vi "Application Memory Monitor.vi"() -> ()   [LabVIEW 2016]
uses:
  <vilib>/Utility/error.llb/DialogType.ctl
  SLL Queued State Machine/Queue Driver/Create Queue.vi
  SLL Queued State Machine/Queue Driver/Enqueue an Item to Queue.vi
  SLL Queued State Machine/Queue Driver/Dequeue Queue.vi
  SLL Queued State Machine/Queue Driver/Enqueue N Items.vi
  SLL Queued State Machine/Queue Driver/Flush Queue.vi
  SLL Queued State Machine/Queue Driver/Release Queue.vi
  SLL Queued State Machine/SLL QSM.lvlib
panel:
  in  "Start":bool
  in  "Sampling Rate (s)":dbl=1.0
  in  "Application Image Name":string="LabVIEW"
  out "Waveform Chart":T1(graph)
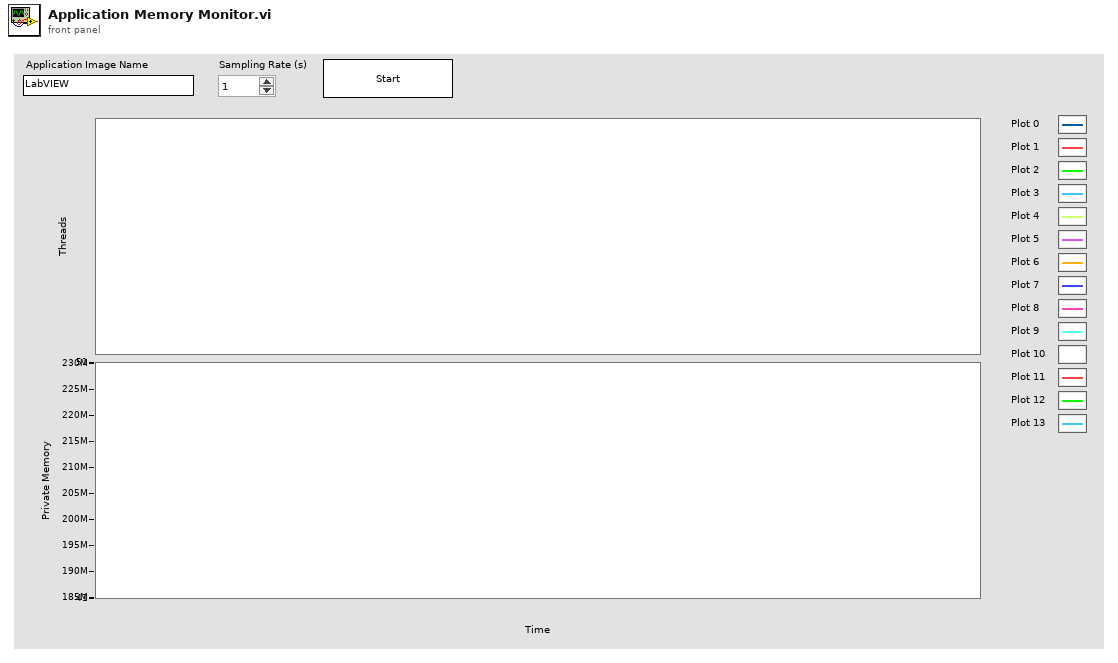
[diagram p1: front panel]
types:
  T1 = cluster{"Thread Count":i32, "PrivateMemorySize64":i64}
  T2 = cluster{"Flags":cluster{"Source Code?":bool, "Running?":bool}, "Application Name":string, "Ref":cluster{"ProcessMain":refnum<k24>, "UserProcess":refnum<k24>, "Threads":refnum<k24>}, "Sampling Rate (ms)":i32}
  T3 = cluster{"Thread Count":i32, "PrivateMemorySize64":i64}[]
  T4 = typedef "DialogType.ctl" = u16
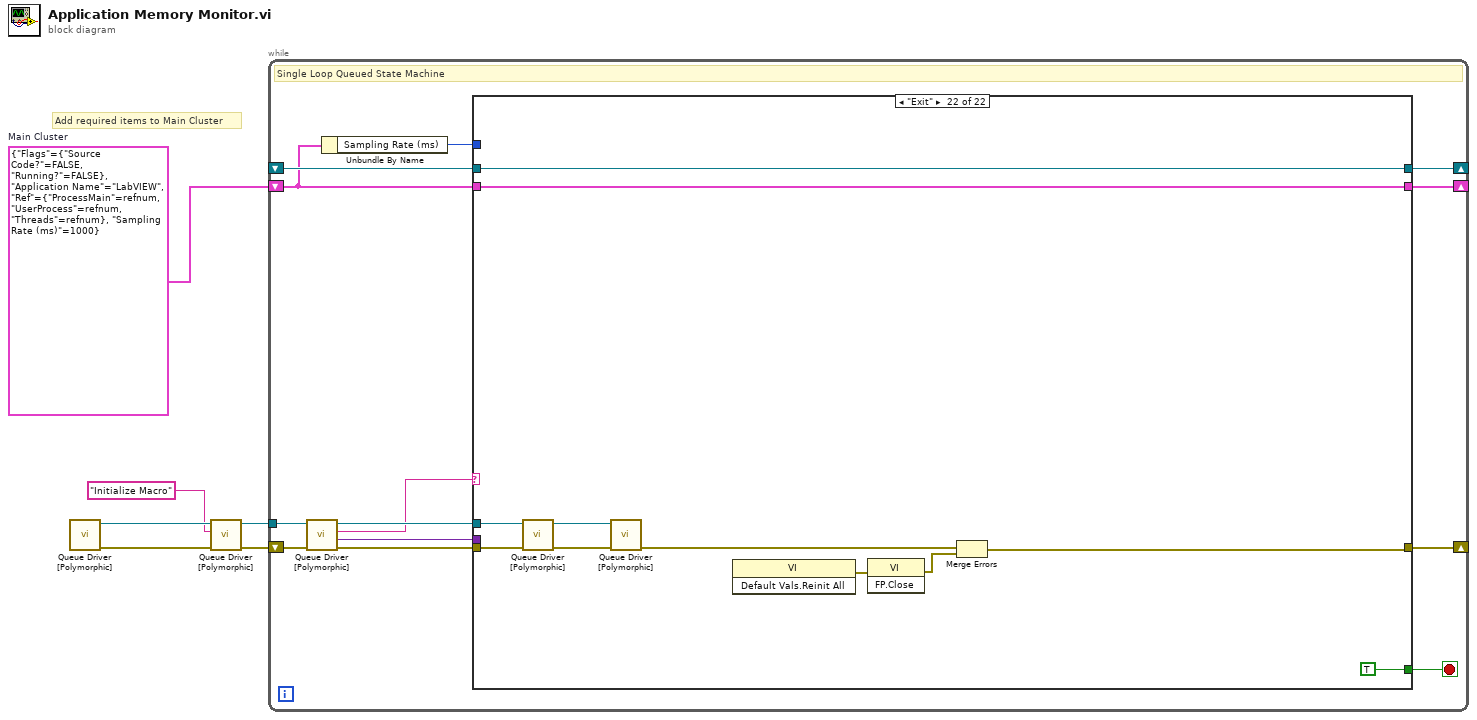
[diagram p0: block diagram]
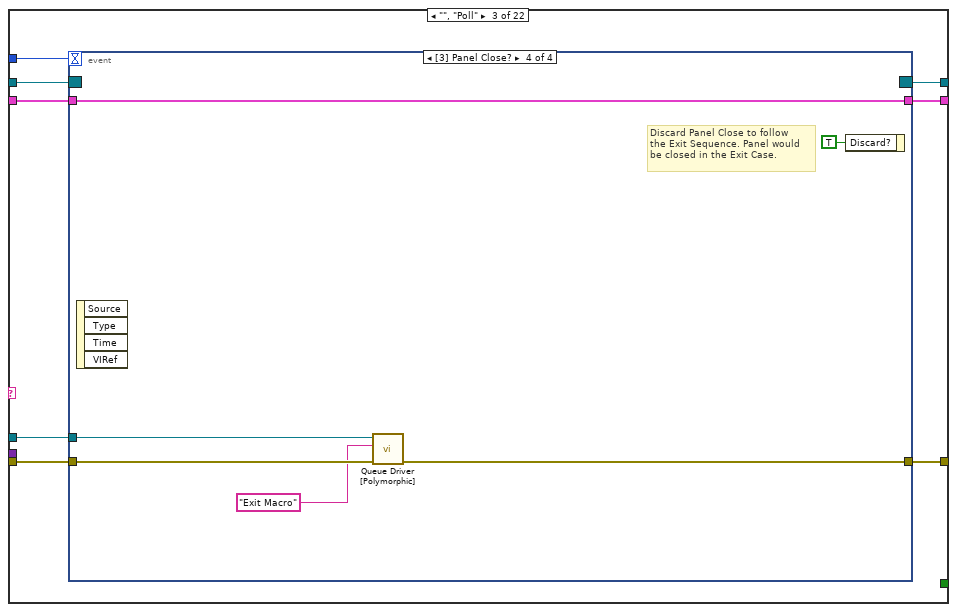
[diagram p4: hidden frame]
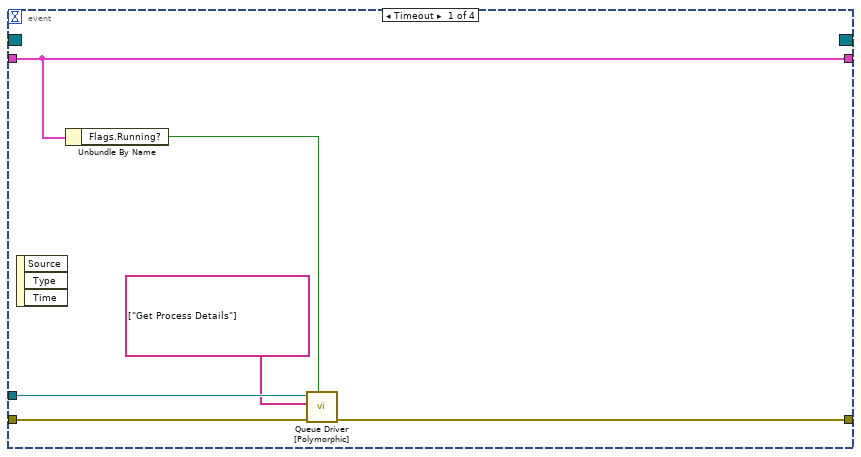
[diagram p5: hidden frame]
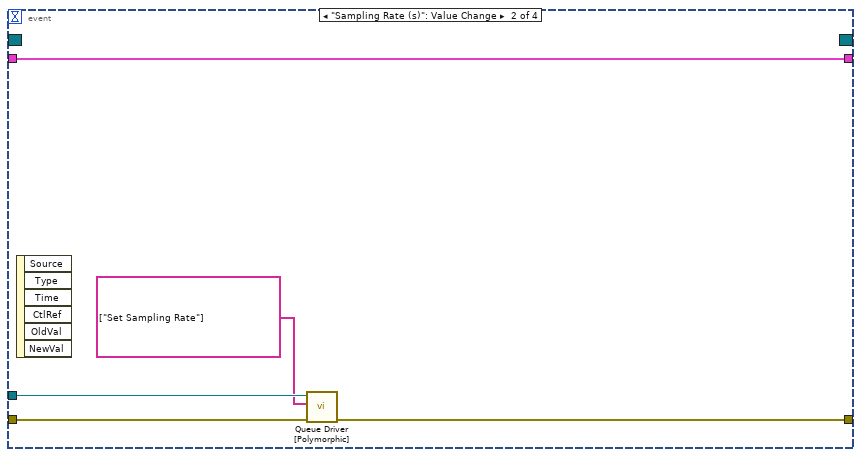
[diagram p6: hidden frame]
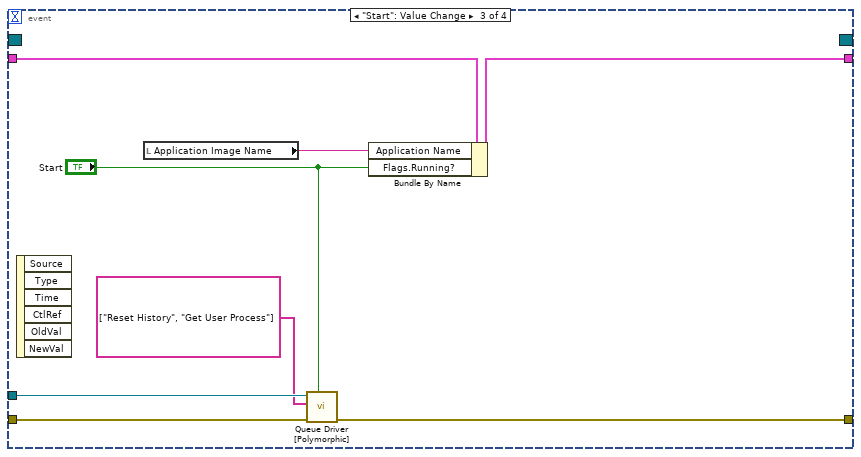
[diagram p7: hidden frame]
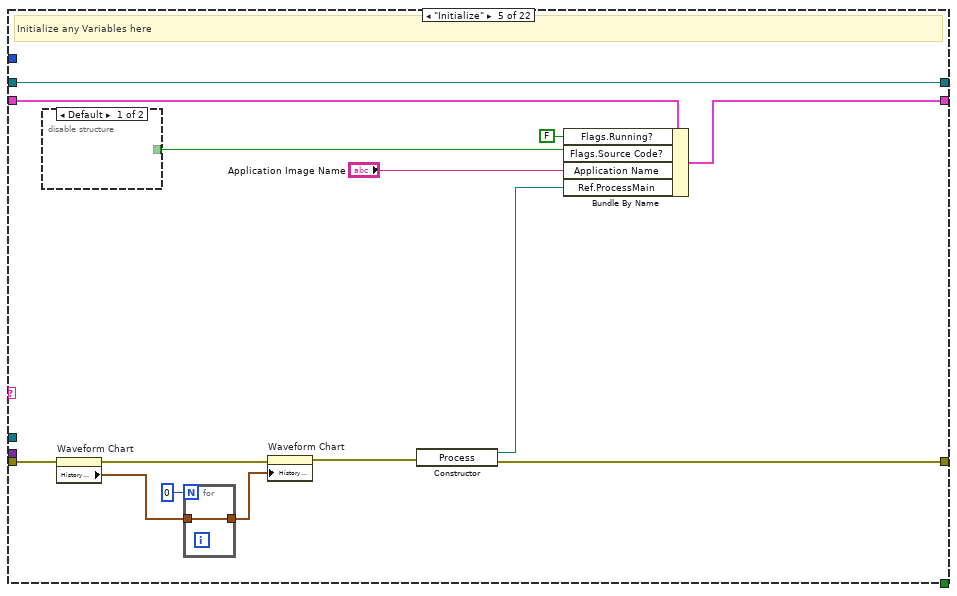
[diagram p9: hidden frame]
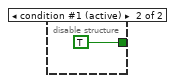
[diagram p10: hidden frame]
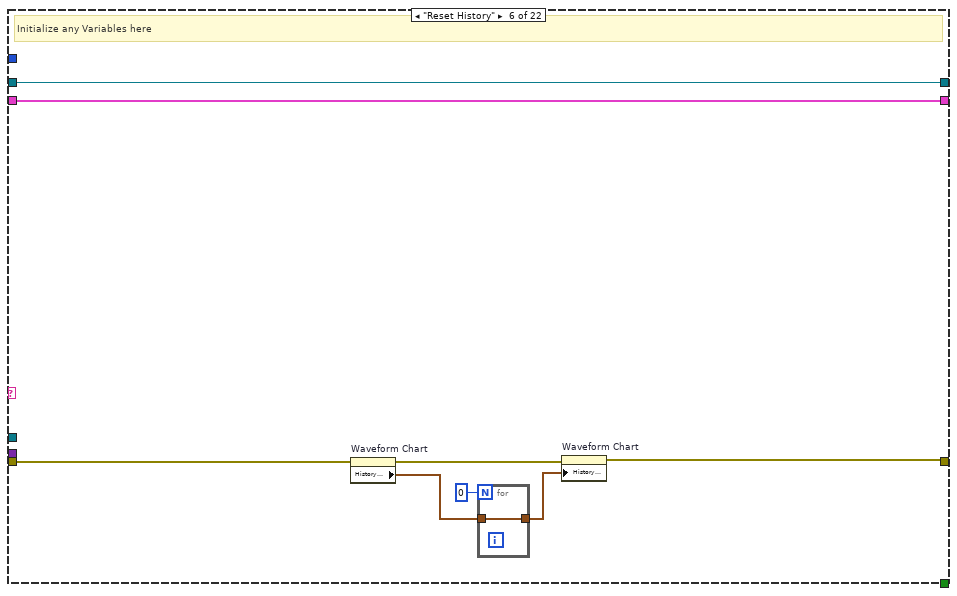
[diagram p11: hidden frame]
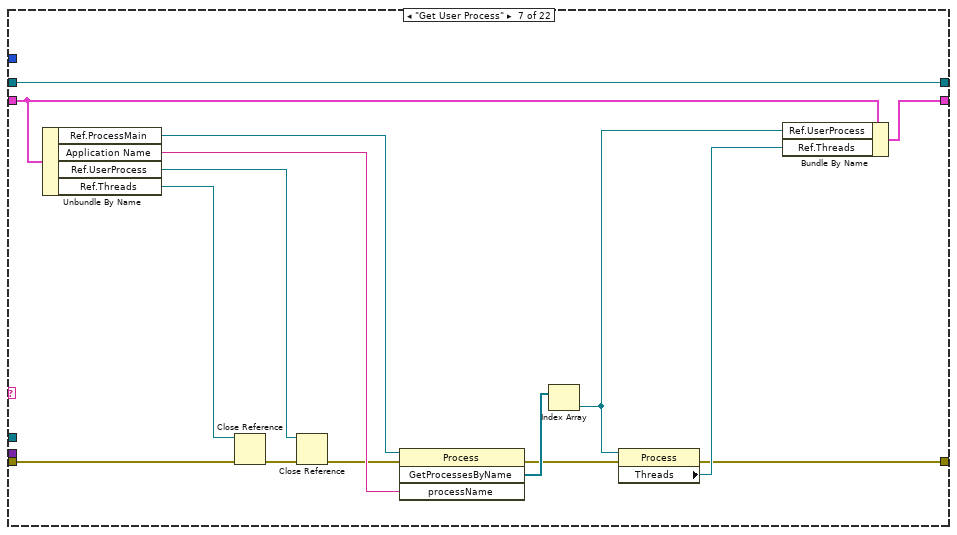
[diagram p12: hidden frame]
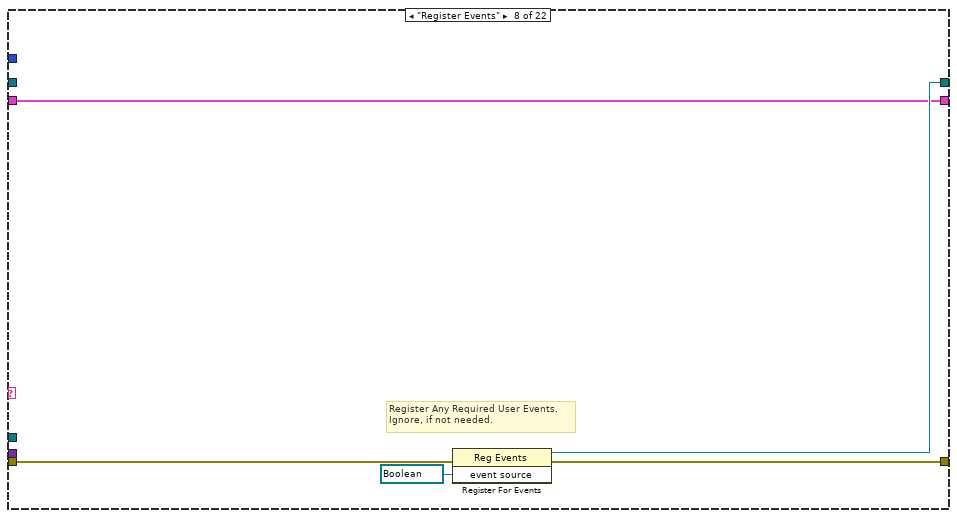
[diagram p13: hidden frame]
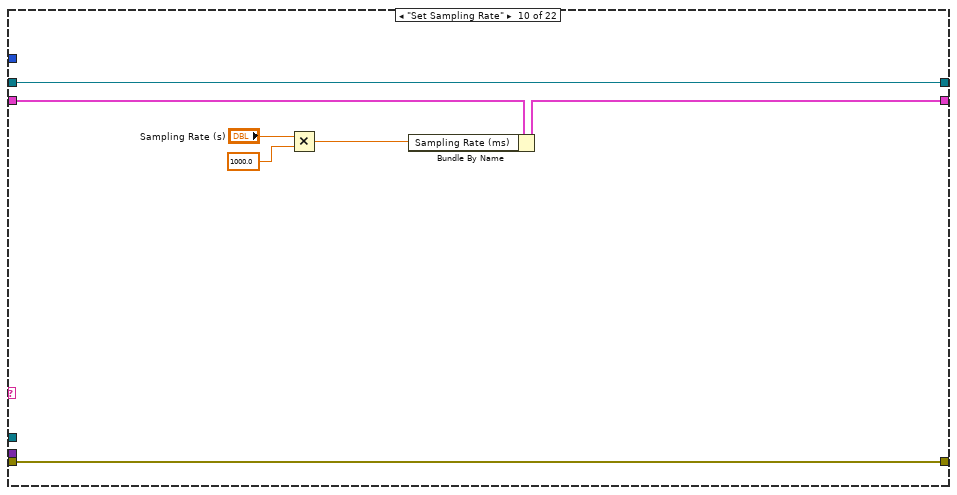
[diagram p15: hidden frame]
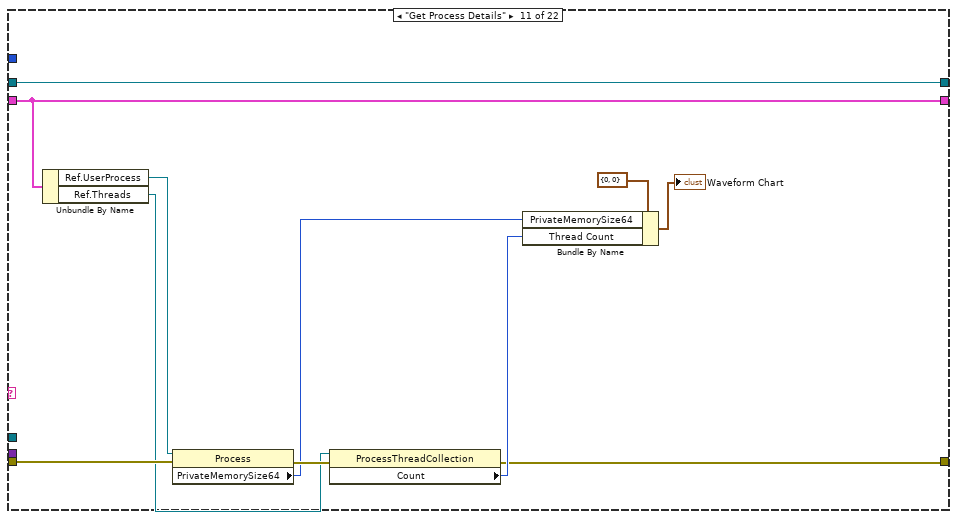
[diagram p16: hidden frame]
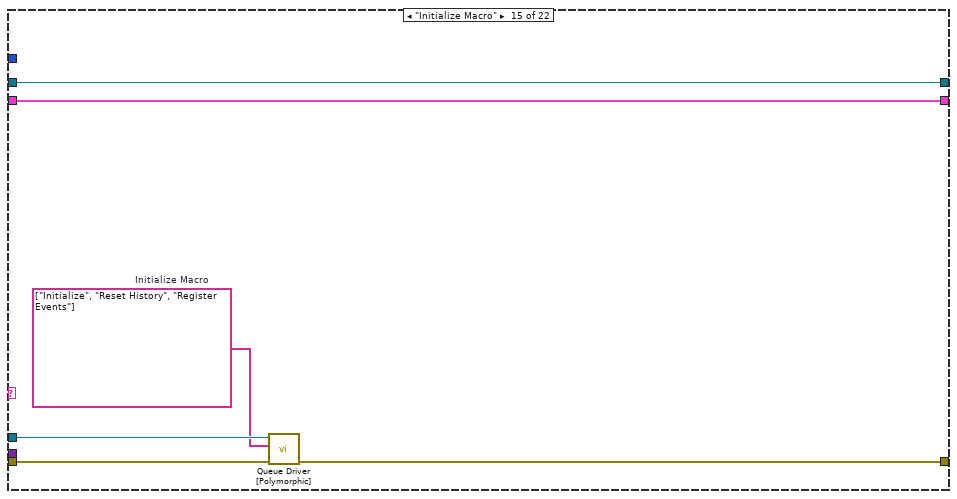
[diagram p20: hidden frame]
diagram:
  w6 = T2 {"Flags"={"Source Code?"=FALSE, "Running?"=FALSE}, "Application Name"="LabVIEW", "Ref"={"ProcessMain"=refnum, "UserProcess"=refnum, "Threads"=refnum}, "Sampling Rate (ms)"=1000}  # Main Cluster
  # "Add required items to Main Cluster"
  n1 = call-poly "Queue Driver [Polymorphic].vi"() -> ("Error Out"=w4:errorcluster, "Queue Ref"=w3:refnum<queue>)  [unwired: 10 in]
  n2 = call-poly "Queue Driver [Polymorphic].vi"("Error In"=w4, "Item to Add"="Initialize Macro", "Queue Ref In"=w3) -> ("Error Out"=w5:errorcluster, "Queue Ref Out"=w1:refnum<queue>)  [unwired: 7 in]
  n3 = while "SLL Queued State Machine" {
    shift-right: [w17] -> _
    shift-left: w5 -> [w19]
    shift-right: [w14] -> _
    shift-left: _ -> [w13]
    shift-right: [w12] -> _
    shift-left: w6 -> [w10]
    tunnel: w1 -> [w8]
    stop <- w16 stop-if-true
    # "Single Loop Queued State Machine"
    n4 = call-poly "Queue Driver [Polymorphic].vi"("Error In"=w19, "Queue Ref In"=w8) -> ("Error Out"=w18:errorcluster, "Data"=w7:variant, "Dequeue"=w11:string, "Queue Ref Out"=w15:refnum<queue>)  [unwired: 6 in]
    n5 = Unbundle By Name(w10) -> ("Sampling Rate (ms)"=w9:i32)
    n6 = case "QSM Case Structure" shown="\"Exit\"" w11 {
      selector: w11 -> [_ _ _ _ _ _ _ _ _ _ _ _ _ _ _ _ _ w152 _ _ _ _]
      tunnel: w18 -> [w22 w25 w32 w61 w68 w83 w98 w106 w109 w116 w125 w130 w133 w136 w140 w146 w151 w155 w167 w170 w174 w188]
      tunnel: [w22 w25 w33 w61 w70 w81 w92 w105 w109 w116 w117 w130 w133 w136 w139 w145 w151 w158 w165 w170 w173 w184] -> w17
      tunnel: [_ _ _ _ _ _ _ _ _ _ _ _ _ _ _ _ _ _ _ _ _ TRUE] -> w16
      tunnel: [w21 w24 w31 w60 w75 w85 w101 w104 w108 w115 w127 w129 w132 w135 w142 w148 w150 w161 w164 w169 w179 w187] -> w14
      tunnel: w13 -> [w21 w24 w30 w60 w75 w85 w101 _ w108 w115 w127 w129 w132 w135 w142 w148 w150 w161 w164 w169 w179 w187]
      tunnel: [w20 w23 w28 w59 w72 w84 w95 w103 w107 w111 w126 w128 w131 w134 w141 w147 w149 w160 w163 w168 w178 w186] -> w12
      tunnel: w10 -> [w20 w23 w29 w59 w73 w84 w96 w103 w107 w114 w126 w128 w131 w134 w141 w147 w149 w160 w163 w168 w178 w186]
      tunnel: w9 -> [_ _ w27 _ _ _ _ _ _ _ _ _ _ _ _ _ _ _ _ _ _ _]
      tunnel: w15 -> [_ _ w26 _ _ _ _ _ _ _ _ _ _ _ w138 w144 _ _ _ _ _ w183]
      tunnel: w7 -> [_ _ _ _ _ _ _ _ _ _ _ _ _ _ _ _ _ _ _ _ _ _]
      frame "/--------------- Read Me -----------------/" {
        # "General Purpose Queue Based State Machine for Any Use Case (main application, module, pop up message etc)\n\nAdvantages:\n1. No Need to Pass Queue References between Queue Driver VIs.\n2. This template can be safely used in multiple parallel running modules without any issues.\n3. This template can also be safely used even in cases where the VI is configured to be a Clone, where multiple \ninstances of the VI could be executing concurrently.\n\nHow to Use:\n1. Add necessary items to the Main Cluster.\n2. Use the Polymorphic Queue Driver for doing any queue operations. There is no need to pass the queue driver\nreference, as the Queue Driver automatically infers the reference based on the VI instance from which it is called.\n3. Add any required user events in the \"Register Events\" case. Ignore if not needed.\n4. Use \"Sequences\" section for defining any list of state calls, which could be used in multiple places. \nExample: Initialize Sequence, might be needed if we need to any reinitialization."
      }
      frame "/------------------ Poll -------------------/" {
      }
      frame "", "Poll" {
        n7 = event shown="[3] Panel Close?" {
          selector: w30 -> [_ _ _ _]
          dyn-events: [_ _ _ _] -> w31
          timeout: w27 -> [_ _ _ _]
          tunnel: [w38 w42 w50 w57] -> w33
          tunnel: w32 -> [w39 w43 w51 w58]
          tunnel: w29 -> [w35 w44 w52 w56]
          tunnel: [w35 w44 w47 w56] -> w28
          tunnel: w26 -> [w37 w41 w49 w53]
          event Timeout {
            n8 = event-data() -> ()  [unwired: 1 in, 3 out]
            n9 = Unbundle By Name(w35) -> ("Flags.Running?"=w34:bool)
            n10 = call-poly "Queue Driver [Polymorphic].vi"("Add to Queue? (T)"=w34, "Error In"=w39, "Enqueue N"=string[] ["Get Process Details"], "Queue Ref In"=w37) -> ("Error Out"=w38:errorcluster)  [unwired: 6 in, 1 out]
          }
          event "Sampling Rate (s)": Value Change {
            n11 = event-data() -> ()  [unwired: 1 in, 6 out]
            n12 = call-poly "Queue Driver [Polymorphic].vi"("Error In"=w43, "Enqueue N"=string[] ["Set Sampling Rate"], "Queue Ref In"=w41) -> ("Error Out"=w42:errorcluster)  [unwired: 7 in, 1 out]
          }
          event "Start": Value Change {
            n13 = event-data() -> ()  [unwired: 1 in, 6 out]
            n14 = local read "Application Image Name"() -> (w45:string)
            n15 = call-poly "Queue Driver [Polymorphic].vi"("Add to Queue? (T)"="Start", "Error In"=w51, "Enqueue N"=string[] ["Reset History", "Get User Process"], "Queue Ref In"=w49) -> ("Error Out"=w50:errorcluster)  [unwired: 6 in, 1 out]
            n16 = Bundle By Name(cluster=w52, "Application Name"=w45, "Flags.Running?"="Start") -> (w47:T2)
          }
          event Panel Close? {
            # "Discard Panel Close to follow\nthe Exit Sequence. Panel would\nbe closed in the Exit Case."
            n17 = event-data() -> ()  [unwired: 1 in, 4 out]
            n18 = call-poly "Queue Driver [Polymorphic].vi"("Error In"=w58, "Item to Add"="Exit Macro" ("Enqueue"), "Queue Ref In"=w53) -> ("Error Out"=w57:errorcluster)  [unwired: 7 in, 1 out]
            n19 = event-data("Discard?"=TRUE) -> ()  [unwired: 1 in, 1 out]
          }
        }
      }
      frame "/--------------- Initialize -----------------/" {
      }
      frame "Initialize" {
        # "Initialize any Variables here"
        n20 = disable-structure shown="Default" {
          disable-tunnel: [_ TRUE] -> w74
          frame condition #0 {
          }
          frame condition #1 (active) {
          }
        }
        n21 = property on="Waveform Chart" class="WFChart (strict)"(error in=w68) -> (error out=w67:errorcluster, "History Data"=w64:T3)  [unwired: 1 in, 1 out]
        n22 = for {
          N: 0 -> [_]
          tunnel: w64 -> [w76]
          tunnel: [w76] -> w63
        }
        n23 = property on="Waveform Chart" class="WFChart (strict)"(error in=w67, "History Data"=w63) -> (error out=w66:errorcluster)  [unwired: 1 in, 1 out]
        n24 = constructor class="Process"(error in=w66) -> (reference out=w69:refnum<k24>, error out=w70:errorcluster)  [unwired: 2 in, 1 out]
        n25 = Bundle By Name(cluster=w73, "Flags.Running?"=FALSE, "Flags.Source Code?"=w74, "Application Name"="Application Image Name", "Ref.ProcessMain"=w69) -> (w72:T2)
      }
      frame "Reset History" {
        # "Initialize any Variables here"
        n26 = property on="Waveform Chart" class="WFChart (strict)"(error in=w83) -> (error out=w82:errorcluster, "History Data"=w79:T3)  [unwired: 1 in, 1 out]
        n27 = for {
          N: 0 -> [_]
          tunnel: w79 -> [w86]
          tunnel: [w86] -> w78
        }
        n28 = property on="Waveform Chart" class="WFChart (strict)"(error in=w82, "History Data"=w78) -> (error out=w81:errorcluster)  [unwired: 1 in, 1 out]
      }
      frame "Get User Process" {
        n29 = Unbundle By Name(w96) -> ("Ref.ProcessMain"=w99:refnum<k24>, "Application Name"=w97:string, "Ref.UserProcess"=w88:refnum<k24>, "Ref.Threads"=w87:refnum<k24>)
        n30 = Close Reference(reference=w87, error in (no error)=w98) -> (error out=w90:errorcluster)
        n31 = Close Reference(reference=w88, error in (no error)=w90) -> (error out=w89:errorcluster)
        n32 = invoke class="Process" method="GetProcessesByName"(reference=w99, error in=w89, "processName"=w97) -> (error out=w91:errorcluster, "GetProcessesByName"=w100:refnum<k24>[])  [unwired: 1 in, 2 out]
        n33 = Index Array(array=w100) -> (element=w94:refnum<k24>)  [unwired: 1 in]
        n34 = property class="Process"(reference=w94, error in=w91) -> (error out=w92:errorcluster, "Threads"=w93:refnum<k24>)  [unwired: 1 out]
        n35 = Bundle By Name(cluster=w96, "Ref.UserProcess"=w94, "Ref.Threads"=w93) -> (w95:T2)
      }
      frame "Register Events" {
        # "Register Any Required User Events. \nIgnore, if not needed."
        n36 = register-events(error in=w106, refnum<vi> refnum ("event source")) -> (reference out=w104:refnum<event-registration>, error out=w105:errorcluster)  [unwired: 1 in]
      }
      frame "/---------- Process Monitor ----------/" {
      }
      frame "Set Sampling Rate" {
        n37 = Multiply(x="Sampling Rate (s)", y=1000.0) -> (x*y=w110:dbl)
        n38 = Bundle By Name(cluster=w114, "Sampling Rate (ms)"=w110) -> (w111:T2)
      }
      frame "Get Process Details" {
        n39 = Unbundle By Name(w126) -> ("Ref.UserProcess"=w124:refnum<k24>, "Ref.Threads"=w121:refnum<k24>)
        n40 = property class="Process"(reference=w124, error in=w125) -> (error out=w123:errorcluster, "PrivateMemorySize64"=w120:i64)  [unwired: 1 out]
        n41 = property class="ProcessThreadCollection"(reference=w121, error in=w123) -> (error out=w117:errorcluster, "Count"=w119:i32)  [unwired: 1 out]
        n42 = Bundle By Name(cluster=T1 {"Thread Count"=0, "PrivateMemorySize64"=0}, "PrivateMemorySize64"=w120, "Thread Count"=w119) -> (→"Waveform Chart":T1)
      }
      frame "/-------------- User Interface --------------/" {
        # "Duplicate this case to create additional case splitters for readability"
      }
      frame "Update UI" {
        # "Update Front Panel Controls in this Case"
      }
      frame "/----------------- Macros -----------------/" {
      }
      frame "Initialize Macro" {
        w137 = string[] ["Initialize", "Reset History", "Register Events"]  # Initialize Macro
        n43 = call-poly "Queue Driver [Polymorphic].vi"("Error In"=w140, "Enqueue N"=w137, "Queue Ref In"=w138) -> ("Error Out"=w139:errorcluster)  [unwired: 7 in, 1 out]
      }
      frame "Exit Macro" {
        n44 = call-poly "Queue Driver [Polymorphic].vi"("Error In"=w146, "Enqueue N"=string[] ["Close References", "Reset History", "Exit"], "Queue Ref In"=w144) -> ("Error Out"=w145:errorcluster)  [unwired: 7 in, 1 out]
      }
      frame "/-------------- Error Handler--------------/" {
      }
      frame Default {
        # "Undefined Case/Spelling Errors - Show Message to Developer"
        n45 = property class="VI"(error in=w155) -> (error out=w154:errorcluster, "Name"=w153:string)  [unwired: 1 in, 1 out]
        n46 = Format Into String(format string="\"%s\" in the VI - %s" ("message"), initial string="Undefined case - ", error in=w154, w152, w153) -> (resulting string=w156:string, error out=w158:errorcluster)
        n47 = One Button Dialog(message=w156) -> ()  [unwired: 1 in, 1 out]
      }
      frame "Error" {
        w162 = T4 2 items=["no dialog", "OK message", "continue or stop message", "OK message + warnings", "continue/stop + warnings"] ("type of dialog (OK msg:1)")
        # "Handle the Error"
        n48 = call <vilib>:"Simple Error Handler.vi"("type of dialog (OK msg:1)"=w162, "error in (no error)"=w167) -> ("error out"=w166:errorcluster)  [unwired: 3 in, 4 out]
        n49 = call <vilib>:"Clear Errors.vi"("error in (no error)"=w166) -> ("error out"=w165:errorcluster)  [unwired: 5 in, 1 out]
      }
      frame "/------------------- Exit --------------------/" {
      }
      frame "Close References" {
        n50 = Unbundle By Name(w178) -> ("Ref.ProcessMain"=w175:refnum<k24>, "Ref.UserProcess"=w176:refnum<k24>, "Ref.Threads"=w171:refnum<k24>)
        n51 = Close Reference(reference=w171, error in (no error)=w174) -> (error out=w172:errorcluster)
        n52 = Close Reference(reference=w176, error in (no error)=w172) -> (error out=w177:errorcluster)
        n53 = Close Reference(reference=w175, error in (no error)=w177) -> (error out=w173:errorcluster)
      }
      frame "Exit" {
        n54 = call-poly "Queue Driver [Polymorphic].vi"("Error In"=w188, "Queue Ref In"=w183) -> ("Error Out"=w189:errorcluster, "Queue Ref Out"=w182:refnum<queue>)  [unwired: 7 in, 1 out]
        n55 = call-poly "Queue Driver [Polymorphic].vi"("Error In"=w189, "Queue Ref In"=w182) -> ("Error Out"=w185:errorcluster)  [unwired: 9 in]
        n56 = invoke class="VI" method="Default Vals.Reinit All"() -> (error out=w180:errorcluster)  [unwired: 3 in, 2 out]
        n57 = invoke class="VI" method="FP.Close"(error in=w180) -> (error out=w181:errorcluster)  [unwired: 2 in, 2 out]
        n58 = Merge Errors(w185, w181) -> (w184:errorcluster)
      }
    }
  }
